vi "Errors.vi"   [LabVIEW 2019, in "DSF Core.lvlib" / "Configuration Session.lvclass"]
uses:
  Configuration Session.lvclass
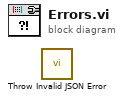
[diagram p0: block diagram]
diagram:
  n1 = call "Throw Invalid JSON Error.vi"() -> ()  [unwired: 11 in, 1 out]
